vi "Speed setup.vi"() -> ()   [LabVIEW 2011]
uses:
  <vilib>/Instr/_visa.llb/VISA Configure Serial Port (Instr).vi
panel:
  out "Error Out":errorcluster={"status"=TRUE, "code"=-1073807343, "source"="VISA Write in Serial Communication for TL3T of VISA.vi"}
  out "concatenated string":string="@0X2000,\r\n"
  in  "Write String":string="@0SI1600,1600,1600"
  in  "baud rate (9600)":u32=9600
  in  "Resource Name 0":refnum<visa-resource-name>="COM3"
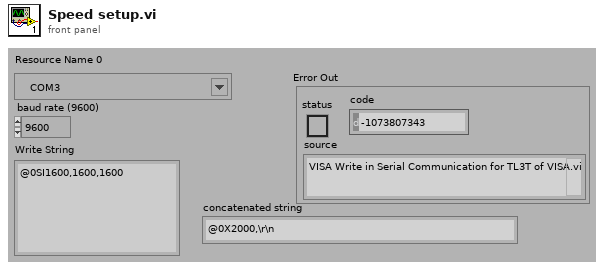
[diagram p1: front panel]
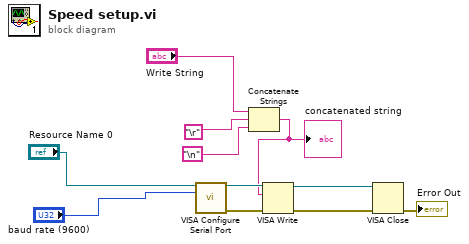
[diagram p0: block diagram]
diagram:
  n1 = call-poly "VISA Configure Serial Port"("VISA resource name"="Resource Name 0", "baud rate (9600)"="baud rate (9600)") -> ("VISA resource name out"=w8:refnum<visa-resource-name>, "error out"=w3:errorcluster)  [unwired: 12 in]
  n2 = Concatenate Strings("Write String", "\r", "\n") -> (w4:string)
  "concatenated string" <- w4
  n3 = VISA Write(VISA resource name=w8, write buffer=w4, error in (no error)=w3) -> (VISA resource name out=w2:refnum<visa-resource-name>, error out=w1:errorcluster)  [unwired: 1 out]
  n4 = VISA Close(VISA resource name=w2, error in (no error)=w1) -> (error out=→"Error Out":errorcluster)
